vi "ReadCalibrationsFromFile.vi"   [LabVIEW 2016]
uses:
  Configurations.vi
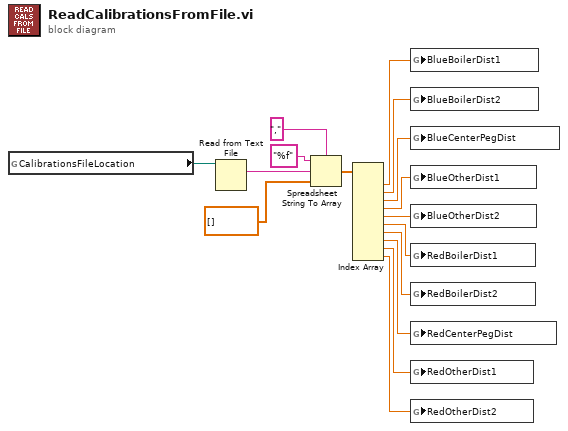
[diagram p0: block diagram]
diagram:
  n1 = global read "Configurations.vi" "CalibrationsFileLocation"() -> (w16:path)
  n2 = Read from Text File(file (use dialog)=w16) -> (text=w15:string)  [unwired: 3 in, 3 out]
  n3 = Spreadsheet String To Array(delimiter (Tab)=",", format string="%f", spreadsheet string=w15, array type (2D Dbl)=dbl[] [] ("appended array")) -> (array=w1:dbl[])
  n4 = Index Array(array=w1) -> (element #1=w11:dbl, element #2=w10:dbl, element #3=w9:dbl, element #4=w8:dbl, element #5=w7:dbl, element #6=w6:dbl, element #7=w5:dbl, element #8=w4:dbl, element #9=w3:dbl, element #10=w2:dbl)  [unwired: 10 in]
  n5 = global write "Configurations.vi" "BlueBoilerDist1"(w11) -> ()
  n6 = global write "Configurations.vi" "BlueBoilerDist2"(w10) -> ()
  n7 = global write "Configurations.vi" "BlueCenterPegDist"(w9) -> ()
  n8 = global write "Configurations.vi" "BlueOtherDist1"(w8) -> ()
  n9 = global write "Configurations.vi" "BlueOtherDist2"(w7) -> ()
  n10 = global write "Configurations.vi" "RedBoilerDist1"(w6) -> ()
  n11 = global write "Configurations.vi" "RedBoilerDist2"(w5) -> ()
  n12 = global write "Configurations.vi" "RedCenterPegDist"(w4) -> ()
  n13 = global write "Configurations.vi" "RedOtherDist1"(w3) -> ()
  n14 = global write "Configurations.vi" "RedOtherDist2"(w2) -> ()
